vi "RSZVB Set Generator Port Trigger Delay.vi"(7 "Trigger Delay (0.0)":dbl format="%^.3e", 8 "error in (no error)":errorcluster {"code" format="%.0x"}, 9 "Generator Port (1)":i32=1, 10 "Channel (1)":i32=1, 11 "VISA session":refnum<visa-resource-name>) -> (0 "error out":errorcluster {"code" format="%.0x"}, 3 "dup VISA session":refnum<visa-resource-name>)   [LabVIEW 2011]
doc: "Defines the trigger delay for a generator port <Gen>. The setting takes effect when a port-specific trigger delay is selected\n\nRemote-control command(s):\nTRIGger<Ch>[:SEQuence]:HOLDoff:GENerator<Gen>"
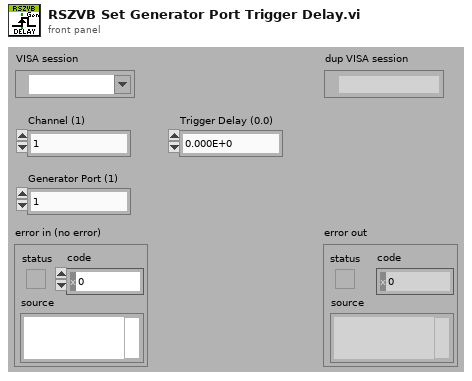
[diagram p1: front panel]
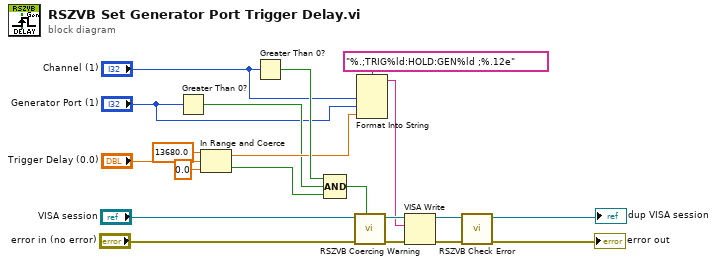
[diagram p0: block diagram]
diagram:
  n1 = Greater Than 0?(x="Generator Port (1)") -> (x > 0?=w2:bool)
  n2 = In Range and Coerce(upper limit=13680.0, x="Trigger Delay (0.0)", lower limit=0.0) -> (coerced(x)=w11:dbl, In Range?=w12:bool)
  n3 = Greater Than 0?(x="Channel (1)") -> (x > 0?=w14:bool)
  n4 = Compound Arithmetic op=AND(w14, w2, w12) -> (w13:bool)
  n5 = call "RSZVB Coercing Warning.vi"("In Range?"=w13, "error in (no error)"="error in (no error)", "VISA session"="VISA session") -> ("error out"=w18:errorcluster, "dup VISA session"=w19:refnum<visa-resource-name>)  [unwired: 7 in]
  n6 = Format Into String(format string="%.;TRIG%ld:HOLD:GEN%ld ;%.12e", "Channel (1)", "Generator Port (1)", w11) -> (resulting string=w15:string)  [unwired: 2 in, 1 out]
  n7 = VISA Write(VISA resource name=w19, write buffer=w15, error in (no error)=w18) -> (VISA resource name out=w16:refnum<visa-resource-name>, error out=w17:errorcluster)  [unwired: 1 out]
  n8 = call "RSZVB Check Error.vi"("error in (no error)"=w17, "VISA session"=w16) -> ("error out"=→"error out":errorcluster, "dup VISA session"=→"dup VISA session":refnum<visa-resource-name>)  [unwired: 8 in]
